vi "Der_ALast.vi"(1 "Y":T1, 2 "A_l":T1) -> (0 "d_AL":T1)   [LabVIEW 2016]
uses:
  <vilib>/Analysis/Matrix/Datatypes/RealMatrix.ctl
  <vilib>/Analysis/Matrix/Numeric/Conversions/Matrix To Array - RM.vi
  <vilib>/Analysis/Matrix/Numeric/Conversions/Array To Matrix - RA2.vi
  <vilib>/Analysis/Matrix/NI_Matrix.lvlib
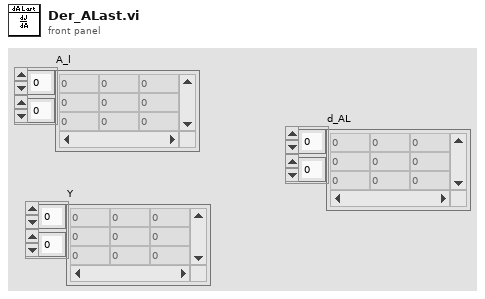
[diagram p1: front panel]
types:
  T1 = typedef "NI_Matrix.lvlib/RealMatrix.ctl" = dbl[][]
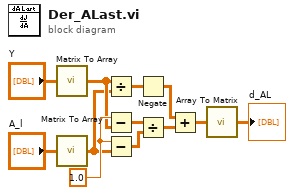
[diagram p0: block diagram]
diagram:
  w9 = 1.0 ("x")
  n1 = call-poly <vilib>:"Matrix To Array.vi"("Real Matrix"="Y") -> ("Real 2D Array"=w8:dbl[][])
  n2 = call-poly <vilib>:"Matrix To Array.vi"("Real Matrix"="A_l") -> ("Real 2D Array"=w7:dbl[][])
  n3 = Divide(x=w8, y=w7) -> (x/y=w10:dbl[][])
  n4 = Subtract(x=w9, y=w8) -> (x-y=w6:dbl[][])
  n5 = Subtract(x=w9, y=w7) -> (x-y=w5:dbl[][])
  n6 = Negate(x=w10) -> (-x=w4:dbl[][])
  n7 = Divide(x=w6, y=w5) -> (x/y=w3:dbl[][])
  n8 = Add(x=w4, y=w3) -> (x+y=w2:dbl[][])
  n9 = call-poly <vilib>:"Array To Matrix.vi"("Real 2D Array"=w2) -> ("Real Matrix"=→"d_AL":T1)
